vi "Begin.vi"(11 "Image Size":T1=enum."160x120") -> (0 "error out":errorcluster)   [LabVIEW 2012]
doc: "Called before other user functions, this VI is expected to open initial I/O refnums, load in file data, and do all program initialization. Notice that the <B>error out</B> terminal is simply used for data flow. Wiring it to other structures or subVIs ensures that this VI runs first."
uses:
  <vilib>/Rock Robotics/WPI/Camera/WPI_CameraImageSize.ctl
  <vilib>/Rock Robotics/WPI/DriverStation/WPI_DriverStationRobotMode2.ctl
  <vilib>/Rock Robotics/WPI/Joystick/WPI_JoystickDeviceEnum.ctl
  <vilib>/Rock Robotics/WPI/CAN/Jaguar/SubVIs/WPI_CANJaguar_ControlMode.ctl
  <vilib>/Rock Robotics/WPI/CAN/Jaguar/SubVIs/WPI_CANJaguar_SpeedReference.ctl
  <vilib>/Rock Robotics/WPI/CAN/Jaguar/SubVIs/WPI_CANJaguar_BrakeCoastMode.ctl
  <vilib>/Rock Robotics/WPI/CAN/Jaguar/SubVIs/WPI_CANJaguar_PositionReference.ctl
  Robot Global Data.vi
  <vilib>/Rock Robotics/WPI/MotorControl/WPI_MotorControlOpenCANJaguar.vi
  <vilib>/Rock Robotics/WPI/Camera/WPI_CameraWhite Balance Values.ctl
  <vilib>/Rock Robotics/WPI/Camera/WPI_CameraExposure Values.ctl
  <vilib>/Rock Robotics/WPI/Camera/WPI_CameraFrameRate.ctl
  <vilib>/Rock Robotics/WPI/RobotDrive/WPI_RobotDriveOpen4MotorWithCANJaguar.vi
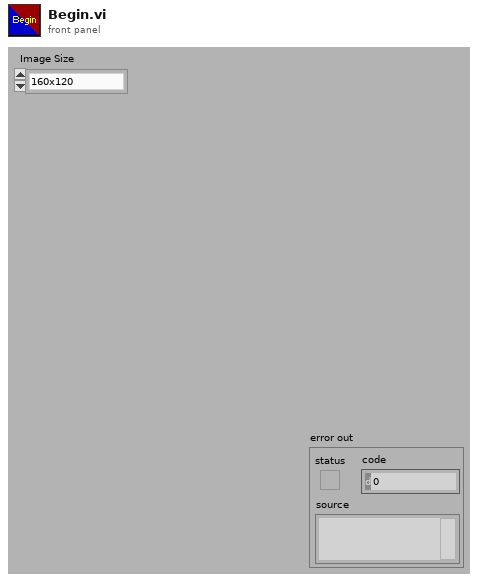
[diagram p1: front panel]
types:
  T1 = typedef "WPI_CameraImageSize.ctl" = enum16{"640x480", "320x240", "160x120"}
  T2 = typedef "WPI_JoystickDeviceEnum.ctl" = enum16{"USB 1", "USB 2", "USB 3", "USB 4", "Kinect 1", "Kinect 2"}
  T3 = typedef "WPI_CANJaguar_PositionReference.ctl" = u8
  T4 = typedef "WPI_CANJaguar_BrakeCoastMode.ctl" = enum8{"Jumper", "Brake", "Coast"}
  T5 = typedef "WPI_CANJaguar_ControlMode.ctl" = enum8{"Percent VBus", "Current", "Speed", "Position", "Voltage"}
  T6 = typedef "WPI_CANJaguar_SpeedReference.ctl" = u8
  T7 = typedef "WPI_DriverStationRobotMode2.ctl" = enum16{"Autonomous Disabled", "Autonomous Enabled", "Teleop Disabled", "Teleop Enabled", "Timeout", "Finish", "Test Disabled", "Test Enabled"}
  T8 = typedef "WPI_JoystickDevRef.ctl" = cluster{"Device":T2}
  T9 = typedef "WPI_SerialPortRef.ctl" = cluster{"DevStatus":errorcluster, "Serial Port Name":refnum<visa-resource-name>}
  T10 = typedef "WPI_CameraFrameRate.ctl" = u32
  T11 = typedef "WPI_CameraExposure Values.ctl" = enum16{"Auto", "Flicker-free 50 Hz", "Flicker-free 60 Hz", "Hold current"}
  T12 = typedef "WPI_CameraWhite Balance Values.ctl" = enum16{"Auto", "Fixed indoor", "Fixed outdoor 1", "Fixed outdoor 2", "Fixed fluorescent 1", "Fixed fluorescent 2", "Hold current"}
  T13 = typedef "WPI_CameraDevRef.ctl" = cluster{"Camera Address":string, "CameraStatus":errorcluster, "Acquire Image Notifier":refnum<notifier>}
  T14 = typedef "WPI_MotorControlDeviceRef.ctl" = cluster{"DeviceStatus":errorcluster, "Type":enum16{"PWM", "CAN"}, "PWM":cluster{"Digital Module":T15, "PWM Channel":T16, "DeadBand":T17}, "CAN":cluster{"Device Number":u8, "Control Mode":T5, "Semaphore":T18, "Max Vout":dbl}, "Invert":bool, "TransformRef":T19, "InvTransformRef":T19}
  T15 = typedef "FPGA_TypedefDigitalModule.ctl" = enum16{"Digital Module 1", "Digital Module 2"}
  T16 = typedef "FPGA_DIOPWMChannel.ctl" = enum8{"PWM 1", "PWM 2", "PWM 3", "PWM 4", "PWM 5", "PWM 6", "PWM 7", "PWM 8", "PWM 9", "PWM 10", "Invalid"}
  T17 = typedef "WPI_PWMDeadband.ctl" = cluster{"Name":string, "maxPositivePwm":i32, "minPositivePwm":i32, "centerPwm":i32, "maxNegativePwm":i32, "minNegativePwm":i32, "angularRange":u16}
  T18 = typedef "Semaphore RefNum" = refnum<k1>
  T19 = typedef "WPI_PWMTransform_ConPane.ctl" = refnum<vi>
  T20 = typedef "WPI_RobotDriveDevRef.ctl" = cluster{"DevStatus":errorcluster, "Motors[]":T14[], "Square Inputs":bool, "Max Output":dbl, "Isochronous":bool}
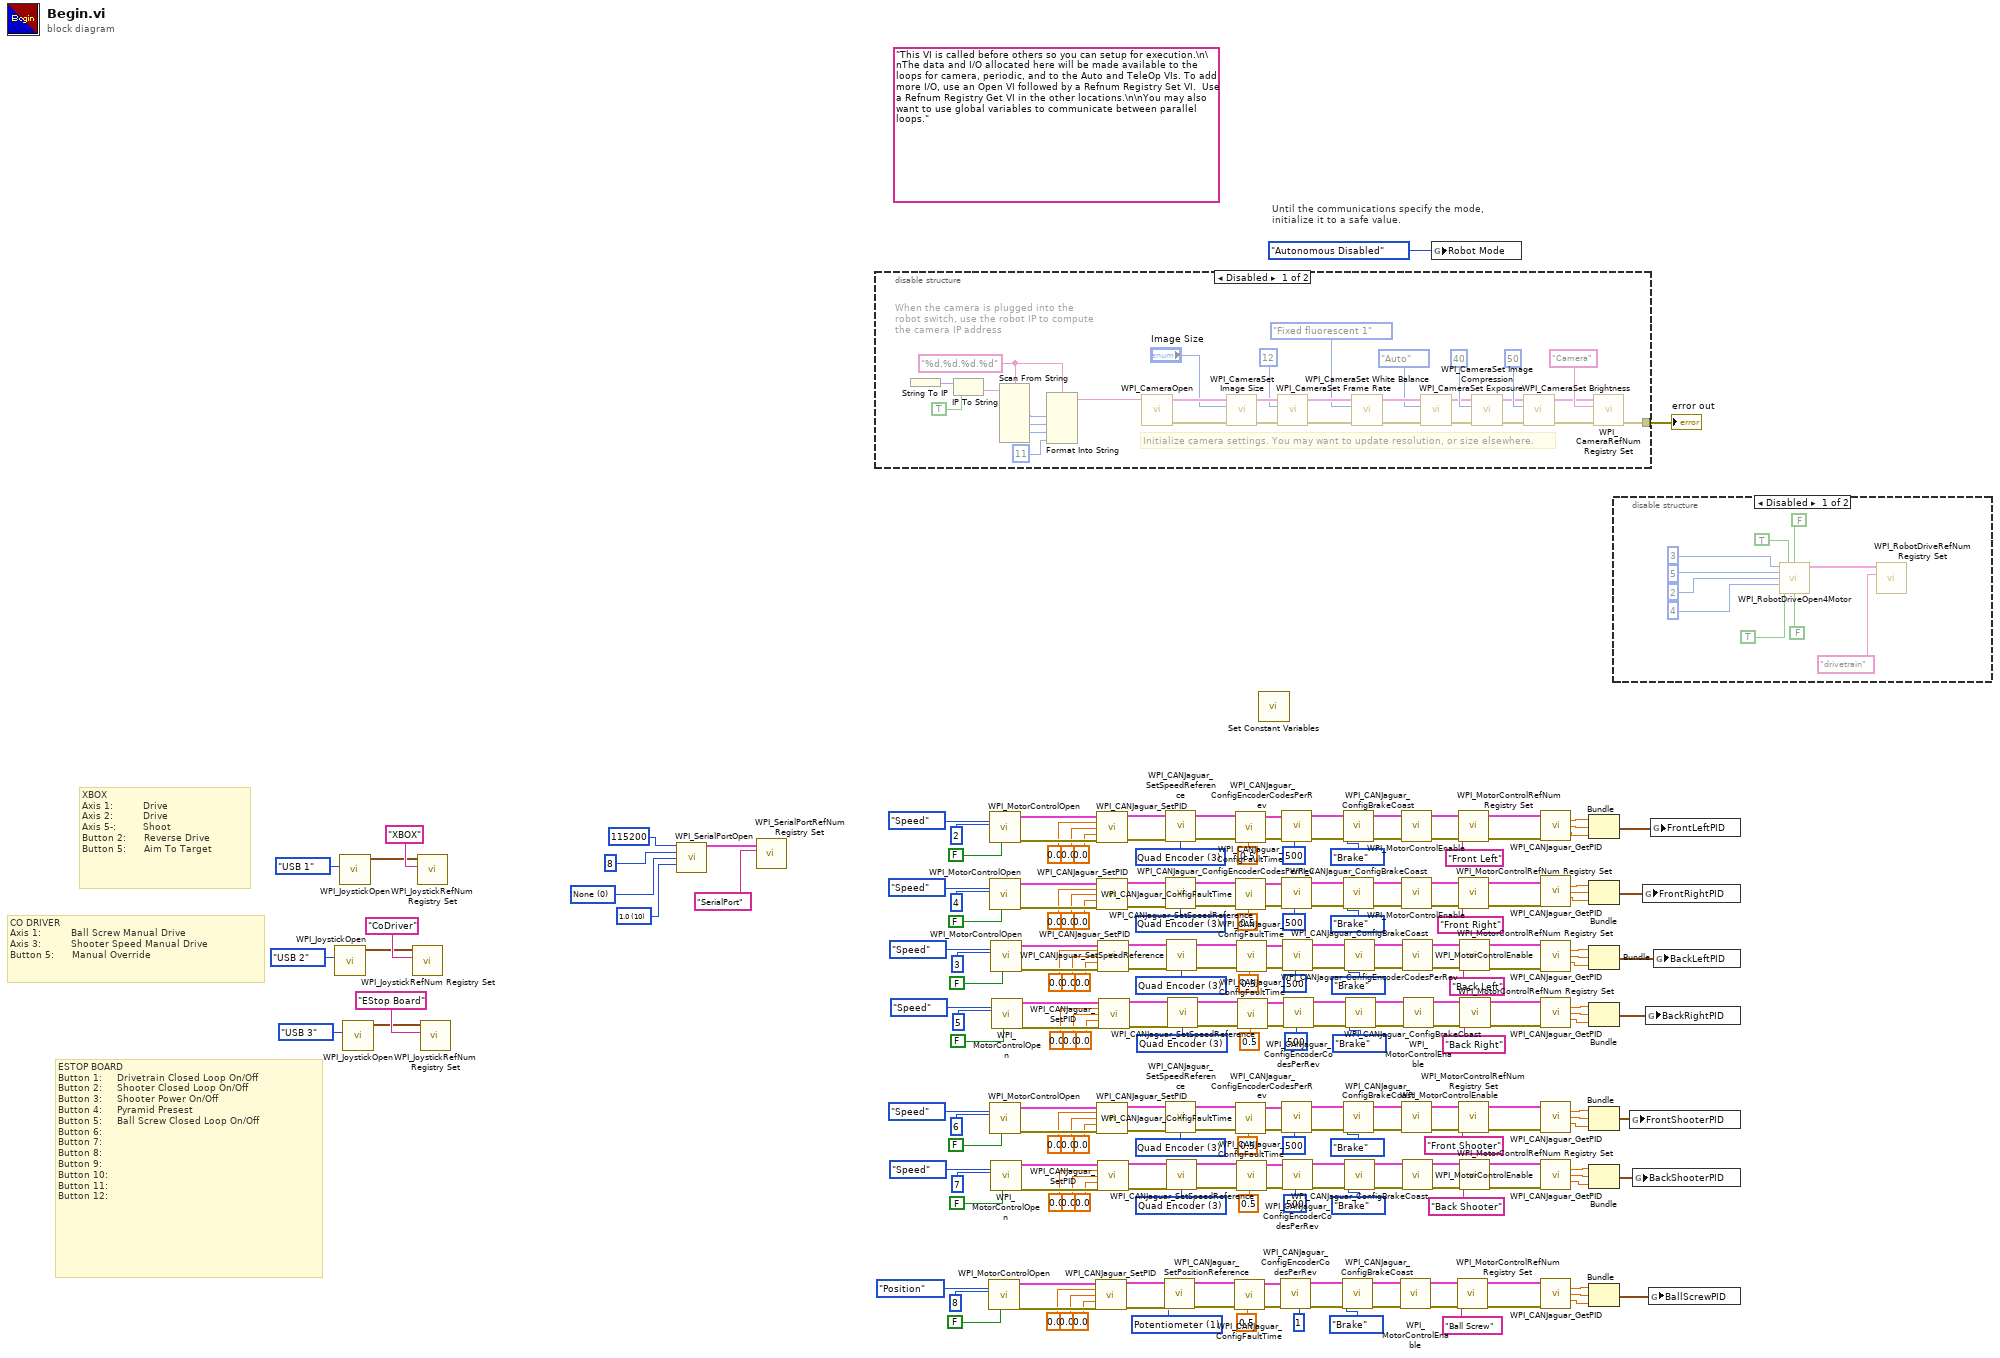
[diagram p0: block diagram]
diagram:
  w49 = T3 1 items=["Quad Encoder"=0, "Potentiometer"=1, "None"=255] ("Position Reference")
  w88 = T6 3 items=["Encoder"=0, "Inv Encoder"=2, "Quad Encoder"=3, "None"=255] ("Speed Reference")
  w113 = T6 3 items=["Encoder"=0, "Inv Encoder"=2, "Quad Encoder"=3, "None"=255] ("Speed Reference")
  w138 = T6 3 items=["Encoder"=0, "Inv Encoder"=2, "Quad Encoder"=3, "None"=255] ("Speed Reference")
  w163 = T6 3 items=["Encoder"=0, "Inv Encoder"=2, "Quad Encoder"=3, "None"=255] ("Speed Reference")
  w188 = T6 3 items=["Encoder"=0, "Inv Encoder"=2, "Quad Encoder"=3, "None"=255] ("Speed Reference")
  w213 = T6 3 items=["Encoder"=0, "Inv Encoder"=2, "Quad Encoder"=3, "None"=255] ("Speed Reference")
  w226 = u16 10 items=["1.0"=10, "1.5"=15, "2.0"=20] ("Stop Bits")
  w227 = u16 0 items=["None", "Odd", "Even", "Mark", "Space"] ("Parity")
  (unwired) "This VI is called before others so you can setup for execution.\n\nThe data and I/O allocated here will be made available to the loops for camera, periodic, and to the Auto and TeleOp VIs. To add more I/O, use an Open VI followed by a Refnum Registry Set VI.  Use a Refnum Registry Get VI in the other locations.\n\nYou may also want to use global variables to communicate between parallel loops."
  # "CO DRIVER\nAxis 1:          Ball Screw Manual Drive\nAxis 3:          Shooter Speed Manual Drive\nButton 5:      Manual Override"
  # "XBOX\nAxis 1:          Drive\nAxis 2:          Drive\nAxis 5-:         Shoot\nButton 2:      Reverse Drive\nButton 5:      Aim To Target"
  # "ESTOP BOARD\nButton 1:     Drivetrain Closed Loop On/Off\nButton 2:     Shooter Closed Loop On/Off\nButton 3:     Shooter Power On/Off\nButton 4:     Pyramid Presest\nButton 5:     Ball Screw Closed Loop On/Off\nButton 6:     \nButton 7:\nButton 8:\nButton 9:\nButton 10:\nButton 11:\nButton 12:"
  # "Until the communications specify the mode,\ninitialize it to a safe value."
  n1 = call <vilib>:"WPI_JoystickOpen.vi"("JoystickDevice"=WPI_JoystickDeviceEnum."USB 2") -> ("JoystickDevRef"=w5:T8)  [unwired: 10 in]
  n2 = call <vilib>:"WPI_JoystickOpen.vi"("JoystickDevice"=WPI_JoystickDeviceEnum."USB 1") -> ("JoystickDevRef"=w232:T8)  [unwired: 10 in]
  n3 = call <vilib>:"WPI_JoystickOpen.vi"("JoystickDevice"=WPI_JoystickDeviceEnum."USB 3") -> ("JoystickDevRef"=w2:T8)  [unwired: 10 in]
  n4 = call <vilib>:"WPI_JoystickRefNum Registry Set.vi"("refnum name"="CoDriver", "JoystickDevRef"=w5) -> ()  [unwired: 8 in, 2 out]
  n5 = call <vilib>:"WPI_JoystickRefNum Registry Set.vi"("refnum name"="XBOX", "JoystickDevRef"=w232) -> ()  [unwired: 8 in, 2 out]
  n6 = call <vilib>:"WPI_JoystickRefNum Registry Set.vi"("refnum name"="EStop Board", "JoystickDevRef"=w2) -> ()  [unwired: 8 in, 2 out]
  n7 = call <vilib>:"WPI_SerialPortOpen.vi"("Baud Rate"=u32 115200, "Data Bits"=u16 8, "Parity"=w227, "Stop Bits"=w226) -> ("SerialPortRef"=w225:T9)  [unwired: 10 in, 1 out]
  n8 = call <vilib>:"WPI_SerialPortRefNum Registry Set.vi"("refnum name"="SerialPort", "SerialPortRef"=w225) -> ()  [unwired: 8 in, 2 out]
  n9 = disable-structure shown="Disabled" {
    disable-tunnel: [w235 _] -> w230
    frame Disabled {
      w237 = "%d.%d.%d.%d" ("format string")
      # "When the camera is plugged into the\nrobot switch, use the robot IP to compute\nthe camera IP address"
      # "Initialize camera settings. You may want to update resolution, or size elsewhere."
      n10 = String To IP() -> (0:w244:u32)  [unwired: 1 in]
      n11 = IP To String(1:TRUE ("dot notation? (F)"), 2:w244) -> (0:w242:string)
      n12 = Scan From String(format string=w237, input string=w242) -> (output 1=w241:i32, output 2=w240:i32, output 3=w239:i32)  [unwired: 7 in, 3 out]
      n13 = Format Into String(format string=w237, w241, w240, w239, 11 ("Compression")) -> (resulting string=w236:string)  [unwired: 2 in, 1 out]
      n14 = call <vilib>:"WPI_CameraOpen.vi"("Camera Address"=w236) -> ("error out"=w256:errorcluster, "CameraDevRef"=w257:T13)  [unwired: 1 in, 8 out]
      n15 = call <vilib>:"WPI_CameraSet Image Size.vi"("error in (no error)"=w256, "Image Size"="Image Size", "CameraDevRef"=w257) -> ("error out"=w255:errorcluster, "CameraDevRef Out"=w258:T13)  [unwired: 7 out]
      n16 = call <vilib>:"WPI_CameraSet Frame Rate.vi"("error in (no error)"=w255, "Frame Rate (fps)"=T10 12, "CameraDevRef"=w258) -> ("error out"=w254:errorcluster, "CameraDevRef Out"=w260:T13)  [unwired: 7 out]
      n17 = call <vilib>:"WPI_CameraSet White Balance.vi"("error in (no error)"=w254, "White Balance"=WPI_CameraWhite_Balance_Values."Fixed fluorescent 1", "CameraDevRef"=w260) -> ("error out"=w253:errorcluster, "CameraDevRef Out"=w259:T13)  [unwired: 7 out]
      n18 = call <vilib>:"WPI_CameraSet Exposure.vi"("error in (no error)"=w253, "Exposure"=WPI_CameraExposure_Values."Auto", "CameraDevRef"=w259) -> ("error out"=w252:errorcluster, "CameraDevRef Out"=w262:T13)  [unwired: 7 out]
      n19 = call <vilib>:"WPI_CameraSet Image Compression.vi"("error in (no error)"=w252, "Compression"=40, "CameraDevRef"=w262) -> ("error out"=w251:errorcluster, "CameraDevRef Out"=w261:T13)  [unwired: 7 out]
      n20 = call <vilib>:"WPI_CameraSet Brightness.vi"("error in (no error)"=w251, "Brightness"=50, "CameraDevRef"=w261) -> ("error out"=w249:errorcluster, "CameraDevRef Out"=w250:T13)  [unwired: 7 out]
      n21 = call <vilib>:"WPI_CameraRefNum Registry Set.vi"("error in (no error)"=w249, "refnum name"="Camera", "CameraDevRef"=w250) -> ("error out"=w235:errorcluster)  [unwired: 8 out]
    }
    frame Enabled {
    }
  }
  "error out" <- w230
  n22 = call-poly <vilib>:"WPI_MotorControlOpen.vi"("Invert"=FALSE, "Device Number"=u8 8, "Control Mode"=WPI_CANJaguar_ControlMode."Position") -> ("error out"=w67:errorcluster, "MotorControlDeviceRef"=w66:T14)  [unwired: 7 in]
  n23 = call-poly <vilib>:"WPI_MotorControlOpen.vi"("Invert"=FALSE, "Device Number"=u8 2, "Control Mode"=WPI_CANJaguar_ControlMode."Speed") -> ("error out"=w217:errorcluster, "MotorControlDeviceRef"=w216:T14)  [unwired: 7 in]
  n24 = call-poly <vilib>:"WPI_MotorControlOpen.vi"("Invert"=FALSE, "Device Number"=u8 4, "Control Mode"=WPI_CANJaguar_ControlMode."Speed") -> ("error out"=w192:errorcluster, "MotorControlDeviceRef"=w191:T14)  [unwired: 7 in]
  n25 = call-poly <vilib>:"WPI_MotorControlOpen.vi"("Invert"=FALSE, "Device Number"=u8 6, "Control Mode"=WPI_CANJaguar_ControlMode."Speed") -> ("error out"=w117:errorcluster, "MotorControlDeviceRef"=w116:T14)  [unwired: 7 in]
  n26 = call-poly <vilib>:"WPI_MotorControlOpen.vi"("Invert"=FALSE, "Device Number"=u8 3, "Control Mode"=WPI_CANJaguar_ControlMode."Speed") -> ("error out"=w167:errorcluster, "MotorControlDeviceRef"=w166:T14)  [unwired: 7 in]
  n27 = call-poly <vilib>:"WPI_MotorControlOpen.vi"("Invert"=FALSE, "Device Number"=u8 7, "Control Mode"=WPI_CANJaguar_ControlMode."Speed") -> ("error out"=w92:errorcluster, "MotorControlDeviceRef"=w91:T14)  [unwired: 7 in]
  n28 = call-poly <vilib>:"WPI_MotorControlOpen.vi"("Invert"=FALSE, "Device Number"=u8 5, "Control Mode"=WPI_CANJaguar_ControlMode."Speed") -> ("error out"=w142:errorcluster, "MotorControlDeviceRef"=w141:T14)  [unwired: 7 in]
  n29 = call <vilib>:"WPI_CANJaguar_SetPID.vi"("CAN Jaguar Ref"=w66, "P"=0.0, "I"=0.0, "D"=0.0, "error in (no error)"=w67) -> ("CAN Jaguar Ref Out"=w73:T14, "error out"=w72:errorcluster)  [unwired: 9 in]
  n30 = call <vilib>:"WPI_CANJaguar_SetPID.vi"("CAN Jaguar Ref"=w216, "P"=0.0, "I"=0.0, "D"=0.0, "error in (no error)"=w217) -> ("CAN Jaguar Ref Out"=w223:T14, "error out"=w222:errorcluster)  [unwired: 9 in]
  n31 = call <vilib>:"WPI_CANJaguar_SetPID.vi"("CAN Jaguar Ref"=w191, "P"=0.0, "I"=0.0, "D"=0.0, "error in (no error)"=w192) -> ("CAN Jaguar Ref Out"=w198:T14, "error out"=w197:errorcluster)  [unwired: 9 in]
  n32 = call <vilib>:"WPI_CANJaguar_SetPID.vi"("CAN Jaguar Ref"=w116, "P"=0.0, "I"=0.0, "D"=0.0, "error in (no error)"=w117) -> ("CAN Jaguar Ref Out"=w123:T14, "error out"=w122:errorcluster)  [unwired: 9 in]
  n33 = call <vilib>:"WPI_CANJaguar_SetPID.vi"("CAN Jaguar Ref"=w166, "P"=0.0, "I"=0.0, "D"=0.0, "error in (no error)"=w167) -> ("CAN Jaguar Ref Out"=w173:T14, "error out"=w172:errorcluster)  [unwired: 9 in]
  n34 = call <vilib>:"WPI_CANJaguar_SetPID.vi"("CAN Jaguar Ref"=w91, "P"=0.0, "I"=0.0, "D"=0.0, "error in (no error)"=w92) -> ("CAN Jaguar Ref Out"=w98:T14, "error out"=w97:errorcluster)  [unwired: 9 in]
  n35 = call <vilib>:"WPI_CANJaguar_SetPID.vi"("CAN Jaguar Ref"=w141, "P"=0.0, "I"=0.0, "D"=0.0, "error in (no error)"=w142) -> ("CAN Jaguar Ref Out"=w148:T14, "error out"=w147:errorcluster)  [unwired: 9 in]
  n36 = call <vilib>:"WPI_CANJaguar_SetPositionReference.vi"("error in (no error)"=w72, "Position Reference"=w49, "CAN Jaguar Ref"=w73) -> ("error out"=w71:errorcluster, "CAN Jaguar Ref Out"=w70:T14)  [unwired: 7 in]
  n37 = call <vilib>:"WPI_CANJaguar_SetSpeedReference.vi"("error in (no error)"=w222, "Speed Reference"=w213, "CAN Jaguar Ref"=w223) -> ("error out"=w221:errorcluster, "CAN Jaguar Ref Out"=w220:T14)  [unwired: 7 in]
  n38 = call <vilib>:"WPI_CANJaguar_SetSpeedReference.vi"("error in (no error)"=w197, "Speed Reference"=w188, "CAN Jaguar Ref"=w198) -> ("error out"=w196:errorcluster, "CAN Jaguar Ref Out"=w195:T14)  [unwired: 7 in]
  n39 = call <vilib>:"WPI_CANJaguar_SetSpeedReference.vi"("error in (no error)"=w122, "Speed Reference"=w113, "CAN Jaguar Ref"=w123) -> ("error out"=w121:errorcluster, "CAN Jaguar Ref Out"=w120:T14)  [unwired: 7 in]
  n40 = call <vilib>:"WPI_CANJaguar_SetSpeedReference.vi"("error in (no error)"=w172, "Speed Reference"=w163, "CAN Jaguar Ref"=w173) -> ("error out"=w171:errorcluster, "CAN Jaguar Ref Out"=w170:T14)  [unwired: 7 in]
  n41 = call <vilib>:"WPI_CANJaguar_SetSpeedReference.vi"("error in (no error)"=w97, "Speed Reference"=w88, "CAN Jaguar Ref"=w98) -> ("error out"=w96:errorcluster, "CAN Jaguar Ref Out"=w95:T14)  [unwired: 7 in]
  n42 = call <vilib>:"WPI_CANJaguar_SetSpeedReference.vi"("error in (no error)"=w147, "Speed Reference"=w138, "CAN Jaguar Ref"=w148) -> ("error out"=w146:errorcluster, "CAN Jaguar Ref Out"=w145:T14)  [unwired: 7 in]
  n43 = call <vilib>:"WPI_CANJaguar_ConfigFaultTime.vi"("error in (no error)"=w71, "Fault Time (s)"=0.5, "CAN Jaguar Ref"=w70) -> ("error out"=w68:errorcluster, "CAN Jaguar Ref Out"=w69:T14)  [unwired: 7 in]
  n44 = call <vilib>:"WPI_CANJaguar_ConfigFaultTime.vi"("error in (no error)"=w221, "Fault Time (s)"=0.5, "CAN Jaguar Ref"=w220) -> ("error out"=w218:errorcluster, "CAN Jaguar Ref Out"=w219:T14)  [unwired: 7 in]
  n45 = call <vilib>:"WPI_CANJaguar_ConfigFaultTime.vi"("error in (no error)"=w196, "Fault Time (s)"=0.5, "CAN Jaguar Ref"=w195) -> ("error out"=w193:errorcluster, "CAN Jaguar Ref Out"=w194:T14)  [unwired: 7 in]
  n46 = call <vilib>:"WPI_CANJaguar_ConfigFaultTime.vi"("error in (no error)"=w121, "Fault Time (s)"=0.5, "CAN Jaguar Ref"=w120) -> ("error out"=w118:errorcluster, "CAN Jaguar Ref Out"=w119:T14)  [unwired: 7 in]
  n47 = call <vilib>:"WPI_CANJaguar_ConfigFaultTime.vi"("error in (no error)"=w171, "Fault Time (s)"=0.5, "CAN Jaguar Ref"=w170) -> ("error out"=w168:errorcluster, "CAN Jaguar Ref Out"=w169:T14)  [unwired: 7 in]
  n48 = call <vilib>:"WPI_CANJaguar_ConfigFaultTime.vi"("error in (no error)"=w96, "Fault Time (s)"=0.5, "CAN Jaguar Ref"=w95) -> ("error out"=w93:errorcluster, "CAN Jaguar Ref Out"=w94:T14)  [unwired: 7 in]
  n49 = call <vilib>:"WPI_CANJaguar_ConfigFaultTime.vi"("error in (no error)"=w146, "Fault Time (s)"=0.5, "CAN Jaguar Ref"=w145) -> ("error out"=w143:errorcluster, "CAN Jaguar Ref Out"=w144:T14)  [unwired: 7 in]
  n50 = call "Set Constant Variables.vi"() -> ()  [unwired: 12 in]
  n51 = call <vilib>:"WPI_CANJaguar_ConfigEncoderCodesPerRev.vi"("error in (no error)"=w68, "Encoder Codes Per Rev"=u16 1, "CAN Jaguar Ref"=w69) -> ("error out"=w61:errorcluster, "CAN Jaguar Ref Out"=w60:T14)  [unwired: 7 in]
  n52 = call <vilib>:"WPI_CANJaguar_ConfigEncoderCodesPerRev.vi"("error in (no error)"=w218, "Encoder Codes Per Rev"=u16 500, "CAN Jaguar Ref"=w219) -> ("error out"=w210:errorcluster, "CAN Jaguar Ref Out"=w209:T14)  [unwired: 7 in]
  n53 = call <vilib>:"WPI_CANJaguar_ConfigEncoderCodesPerRev.vi"("error in (no error)"=w193, "Encoder Codes Per Rev"=u16 500, "CAN Jaguar Ref"=w194) -> ("error out"=w185:errorcluster, "CAN Jaguar Ref Out"=w184:T14)  [unwired: 7 in]
  n54 = call <vilib>:"WPI_CANJaguar_ConfigEncoderCodesPerRev.vi"("error in (no error)"=w118, "Encoder Codes Per Rev"=u16 500, "CAN Jaguar Ref"=w119) -> ("error out"=w110:errorcluster, "CAN Jaguar Ref Out"=w109:T14)  [unwired: 7 in]
  n55 = call <vilib>:"WPI_CANJaguar_ConfigEncoderCodesPerRev.vi"("error in (no error)"=w168, "Encoder Codes Per Rev"=u16 500, "CAN Jaguar Ref"=w169) -> ("error out"=w160:errorcluster, "CAN Jaguar Ref Out"=w159:T14)  [unwired: 7 in]
  n56 = call <vilib>:"WPI_CANJaguar_ConfigEncoderCodesPerRev.vi"("error in (no error)"=w93, "Encoder Codes Per Rev"=u16 500, "CAN Jaguar Ref"=w94) -> ("error out"=w85:errorcluster, "CAN Jaguar Ref Out"=w84:T14)  [unwired: 7 in]
  n57 = call <vilib>:"WPI_CANJaguar_ConfigEncoderCodesPerRev.vi"("error in (no error)"=w143, "Encoder Codes Per Rev"=u16 500, "CAN Jaguar Ref"=w144) -> ("error out"=w135:errorcluster, "CAN Jaguar Ref Out"=w134:T14)  [unwired: 7 in]
  n58 = call <vilib>:"WPI_CANJaguar_ConfigBrakeCoast.vi"("error in (no error)"=w61, "Brake / Coast Mode"=WPI_CANJaguar_BrakeCoastMode."Brake", "CAN Jaguar Ref"=w60) -> ("error out"=w52:errorcluster, "CAN Jaguar Ref Out"=w53:T14)  [unwired: 7 in]
  n59 = call <vilib>:"WPI_CANJaguar_ConfigBrakeCoast.vi"("error in (no error)"=w210, "Brake / Coast Mode"=WPI_CANJaguar_BrakeCoastMode."Brake", "CAN Jaguar Ref"=w209) -> ("error out"=w201:errorcluster, "CAN Jaguar Ref Out"=w202:T14)  [unwired: 7 in]
  n60 = call <vilib>:"WPI_CANJaguar_ConfigBrakeCoast.vi"("error in (no error)"=w185, "Brake / Coast Mode"=WPI_CANJaguar_BrakeCoastMode."Brake", "CAN Jaguar Ref"=w184) -> ("error out"=w176:errorcluster, "CAN Jaguar Ref Out"=w177:T14)  [unwired: 7 in]
  n61 = call <vilib>:"WPI_CANJaguar_ConfigBrakeCoast.vi"("error in (no error)"=w110, "Brake / Coast Mode"=WPI_CANJaguar_BrakeCoastMode."Brake", "CAN Jaguar Ref"=w109) -> ("error out"=w101:errorcluster, "CAN Jaguar Ref Out"=w102:T14)  [unwired: 7 in]
  n62 = call <vilib>:"WPI_CANJaguar_ConfigBrakeCoast.vi"("error in (no error)"=w160, "Brake / Coast Mode"=WPI_CANJaguar_BrakeCoastMode."Brake", "CAN Jaguar Ref"=w159) -> ("error out"=w151:errorcluster, "CAN Jaguar Ref Out"=w152:T14)  [unwired: 7 in]
  n63 = call <vilib>:"WPI_CANJaguar_ConfigBrakeCoast.vi"("error in (no error)"=w85, "Brake / Coast Mode"=WPI_CANJaguar_BrakeCoastMode."Brake", "CAN Jaguar Ref"=w84) -> ("error out"=w76:errorcluster, "CAN Jaguar Ref Out"=w77:T14)  [unwired: 7 in]
  n64 = call <vilib>:"WPI_CANJaguar_ConfigBrakeCoast.vi"("error in (no error)"=w135, "Brake / Coast Mode"=WPI_CANJaguar_BrakeCoastMode."Brake", "CAN Jaguar Ref"=w134) -> ("error out"=w126:errorcluster, "CAN Jaguar Ref Out"=w127:T14)  [unwired: 7 in]
  n65 = call <vilib>:"WPI_MotorControlEnable.vi"("error in (no error)"=w52, "CAN Jaguar Ref"=w53) -> ("error out"=w50:errorcluster, "CAN Jaguar Ref Out"=w51:T14)  [unwired: 8 in]
  n66 = call <vilib>:"WPI_MotorControlEnable.vi"("error in (no error)"=w201, "CAN Jaguar Ref"=w202) -> ("error out"=w199:errorcluster, "CAN Jaguar Ref Out"=w200:T14)  [unwired: 8 in]
  n67 = call <vilib>:"WPI_MotorControlEnable.vi"("error in (no error)"=w176, "CAN Jaguar Ref"=w177) -> ("error out"=w174:errorcluster, "CAN Jaguar Ref Out"=w175:T14)  [unwired: 8 in]
  n68 = call <vilib>:"WPI_MotorControlEnable.vi"("error in (no error)"=w101, "CAN Jaguar Ref"=w102) -> ("error out"=w99:errorcluster, "CAN Jaguar Ref Out"=w100:T14)  [unwired: 8 in]
  n69 = call <vilib>:"WPI_MotorControlEnable.vi"("error in (no error)"=w151, "CAN Jaguar Ref"=w152) -> ("error out"=w149:errorcluster, "CAN Jaguar Ref Out"=w150:T14)  [unwired: 8 in]
  n70 = call <vilib>:"WPI_MotorControlEnable.vi"("error in (no error)"=w76, "CAN Jaguar Ref"=w77) -> ("error out"=w74:errorcluster, "CAN Jaguar Ref Out"=w75:T14)  [unwired: 8 in]
  n71 = call <vilib>:"WPI_MotorControlEnable.vi"("error in (no error)"=w126, "CAN Jaguar Ref"=w127) -> ("error out"=w124:errorcluster, "CAN Jaguar Ref Out"=w125:T14)  [unwired: 8 in]
  n72 = global write "Robot Global Data.vi" "Robot Mode"(WPI_DriverStationRobotMode2."Autonomous Disabled" ("Robot Mode")) -> ()
  n73 = call <vilib>:"WPI_MotorControlRefNum Registry Set.vi"("error in (no error)"=w50, "refnum name"="Ball Screw", "MotorControlDevRef"=w51) -> ("error out"=w7:errorcluster, "MotorControlDevRef"=w8:T14)  [unwired: 7 in]
  n74 = call <vilib>:"WPI_MotorControlRefNum Registry Set.vi"("error in (no error)"=w199, "refnum name"="Front Left", "MotorControlDevRef"=w200) -> ("error out"=w32:errorcluster, "MotorControlDevRef"=w48:T14)  [unwired: 7 in]
  n75 = call <vilib>:"WPI_MotorControlRefNum Registry Set.vi"("error in (no error)"=w174, "refnum name"="Front Right", "MotorControlDevRef"=w175) -> ("error out"=w33:errorcluster, "MotorControlDevRef"=w34:T14)  [unwired: 7 in]
  n76 = call <vilib>:"WPI_MotorControlRefNum Registry Set.vi"("error in (no error)"=w99, "refnum name"="Front Shooter", "MotorControlDevRef"=w100) -> ("error out"=w11:errorcluster, "MotorControlDevRef"=w12:T14)  [unwired: 7 in]
  n77 = call <vilib>:"WPI_MotorControlRefNum Registry Set.vi"("error in (no error)"=w149, "refnum name"="Back Left", "MotorControlDevRef"=w150) -> ("error out"=w31:errorcluster, "MotorControlDevRef"=w39:T14)  [unwired: 7 in]
  n78 = call <vilib>:"WPI_MotorControlRefNum Registry Set.vi"("error in (no error)"=w74, "refnum name"="Back Shooter", "MotorControlDevRef"=w75) -> ("error out"=w9:errorcluster, "MotorControlDevRef"=w10:T14)  [unwired: 7 in]
  n79 = call <vilib>:"WPI_MotorControlRefNum Registry Set.vi"("error in (no error)"=w124, "refnum name"="Back Right", "MotorControlDevRef"=w125) -> ("error out"=w25:errorcluster, "MotorControlDevRef"=w26:T14)  [unwired: 7 in]
  n80 = call <vilib>:"WPI_CANJaguar_GetPID.vi"("CAN Jaguar Ref"=w48, "error in (no error)"=w32) -> ("P"=w46:dbl, "I"=w44:dbl, "D"=w45:dbl)  [unwired: 9 in, 2 out]
  n81 = call <vilib>:"WPI_CANJaguar_GetPID.vi"("CAN Jaguar Ref"=w34, "error in (no error)"=w33) -> ("P"=w37:dbl, "I"=w35:dbl, "D"=w36:dbl)  [unwired: 9 in, 2 out]
  n82 = call <vilib>:"WPI_CANJaguar_GetPID.vi"("CAN Jaguar Ref"=w39, "error in (no error)"=w31) -> ("P"=w42:dbl, "I"=w40:dbl, "D"=w41:dbl)  [unwired: 9 in, 2 out]
  n83 = call <vilib>:"WPI_CANJaguar_GetPID.vi"("CAN Jaguar Ref"=w26, "error in (no error)"=w25) -> ("P"=w29:dbl, "I"=w27:dbl, "D"=w28:dbl)  [unwired: 9 in, 2 out]
  n84 = call <vilib>:"WPI_CANJaguar_GetPID.vi"("CAN Jaguar Ref"=w12, "error in (no error)"=w11) -> ("P"=w23:dbl, "I"=w21:dbl, "D"=w22:dbl)  [unwired: 9 in, 2 out]
  n85 = call <vilib>:"WPI_CANJaguar_GetPID.vi"("CAN Jaguar Ref"=w10, "error in (no error)"=w9) -> ("P"=w19:dbl, "I"=w17:dbl, "D"=w18:dbl)  [unwired: 9 in, 2 out]
  n86 = call <vilib>:"WPI_CANJaguar_GetPID.vi"("CAN Jaguar Ref"=w8, "error in (no error)"=w7) -> ("P"=w15:dbl, "I"=w13:dbl, "D"=w14:dbl)  [unwired: 9 in, 2 out]
  n87 = Bundle("P"=w46, "I"=w44, "D"=w45) -> (w47:cluster{"P":dbl, "I":dbl, "D":dbl})  [unwired: 1 in]
  n88 = Bundle("P"=w37, "I"=w35, "D"=w36) -> (w38:cluster{"P":dbl, "I":dbl, "D":dbl})  [unwired: 1 in]
  n89 = Bundle("P"=w42, "I"=w40, "D"=w41) -> (w43:cluster{"P":dbl, "I":dbl, "D":dbl})  [unwired: 1 in]
  n90 = Bundle("P"=w29, "I"=w27, "D"=w28) -> (w30:cluster{"P":dbl, "I":dbl, "D":dbl})  [unwired: 1 in]
  n91 = Bundle("P"=w23, "I"=w21, "D"=w22) -> (w24:cluster{"P":dbl, "I":dbl, "D":dbl})  [unwired: 1 in]
  n92 = Bundle("P"=w19, "I"=w17, "D"=w18) -> (w20:cluster{"P":dbl, "I":dbl, "D":dbl})  [unwired: 1 in]
  n93 = Bundle("P"=w15, "I"=w13, "D"=w14) -> (w16:cluster{"P":dbl, "I":dbl, "D":dbl})  [unwired: 1 in]
  n94 = disable-structure shown="Disabled" {
    frame Disabled {
      n95 = call-poly <vilib>:"WPI_RobotDriveOpen4Motor.vi"("Rear Left Motor"=u8 3, "Rear Left Motor Inverted"=TRUE, "Rear Right Motor Inverted"=FALSE, "Rear Right Motor"=u8 5 ("Rear Left Motor"), "Front Left Motor"=u8 2 ("Rear Left Motor"), "Front Right Motor"=u8 4 ("Rear Left Motor"), "Front Left Motor Inverted"=TRUE, "Front Right Motor Inverted"=FALSE) -> ("RobotDriveDevRef"=w267:T20)  [unwired: 6 in, 1 out]
      n96 = call <vilib>:"WPI_RobotDriveRefNum Registry Set.vi"("refnum name"="drivetrain", "RobotDriveDevRef"=w267) -> ()  [unwired: 8 in, 2 out]
    }
    frame Enabled {
    }
  }
  n97 = global write "Robot Global Data.vi" "FrontShooterPID"(w24) -> ()
  n98 = global write "Robot Global Data.vi" "BackShooterPID"(w20) -> ()
  n99 = global write "Robot Global Data.vi" "FrontRightPID"(w38) -> ()
  n100 = global write "Robot Global Data.vi" "BackRightPID"(w30) -> ()
  n101 = global write "Robot Global Data.vi" "BallScrewPID"(w16) -> ()
  n102 = global write "Robot Global Data.vi" "FrontLeftPID"(w47) -> ()
  n103 = global write "Robot Global Data.vi" "BackLeftPID"(w43) -> ()
